vi "pid-tuning-v2.vi"() -> ()   [LabVIEW 2019]
uses:
  <vilib>/DAQmx/read.llb/DAQmx Read (Analog 1D DBL 1Chan NSamp).vi
  <vilib>/Analysis/baseanly.llb/Mean (DBL).vi
  <vilib>/DAQmx/write.llb/DAQmx Write (Analog DBL 1Chan 1Samp).vi
  <vilib>/DAQmx/create/channels.llb/DAQmx Create Channel (AO-Current-Basic).vi
  <vilib>/DAQmx/create/channels.llb/DAQmx Create Channel (AI-Current-Basic).vi
  <vilib>/DAQmx/miscellaneous.llb/DAQmx Fill In Error Info.vi
  <vilib>/Analysis/NI_AALBase.lvlib
  <vilib>/addons/control/pid/NI_PID_autopid.lvlib
panel:
  out "PID FINAL POWER":dbl
  in  "stop":bool
  out "PID START TIME":dbl
  in  "Tabs":T1(tab)
  in  "POWER CONTROL":dbl format="%#_13g"
  in  "ENABLE FURNACE TEST":bool[](array[boolean])=[FALSE]
  in  "STOP FURNACE TEST":bool[](array[boolean])=[FALSE]
  in  "Close Valve":bool[](array[boolean])=[TRUE]
  in  "Purge Flow":bool[](array[boolean])=[FALSE]
  in  "ARGON OUT 0-.02":dbl format="%#_13g"
  out "VALVE OUTPUT":dbl
  out "PYROMETER TEMP":dbl
  out "PYROMETER READING":dbl
  in  "RAMP UP POWER":dbl format="%#_13g"
  out "TEMPERATURE OVER TIME":cluster{dbl[], dbl[]}[](graph)
  out "CURRENT TEMPERATURE (C)":dbl
  in  "PID SETPOINT":dbl=820.0
  in  "Clear Data":bool
  in  "Restart PID":bool
  in  "PID gains":T2={"proportional gain (Kc)"=5e-05, "integral time (Ti, min)"=1.5, "derivative time (Td, min)"=0.0} {"derivative time (Td, min)" format="%.8f"; "integral time (Ti, min)" format="%.24f"; "proportional gain (Kc)" format="%.8f"}
  out "POWER LEVEL OUTPUT (%)":dbl
  out "tuning completed?":bool
  in  "autotune? (F)":bool
  out "PID gains out":T2={"proportional gain (Kc)"=1.0, "integral time (Ti, min)"=0.01, "derivative time (Td, min)"=0.0} {"derivative time (Td, min)" format="%.3f"; "integral time (Ti, min)" format="%.3f"; "proportional gain (Kc)" format="%.3f"}
  out "Time has Elapsed 2":bool caption="Time has Elapsed"
  out "CURRENT RAMP DOWN POWER LEVEL":string
  out "PYROMETER READING 2":dbl
  in  "RAMP DOWN TIME (min)":dbl=10.0
  in  "Mode":T3(ring)
  in  "POWER OUT":dbl format="%#_13g"
  in  "STOP FURNACE":bool[](array[boolean])
  in  "ENABLE FURNACE":bool[](array[boolean])
  out "DONE":bool
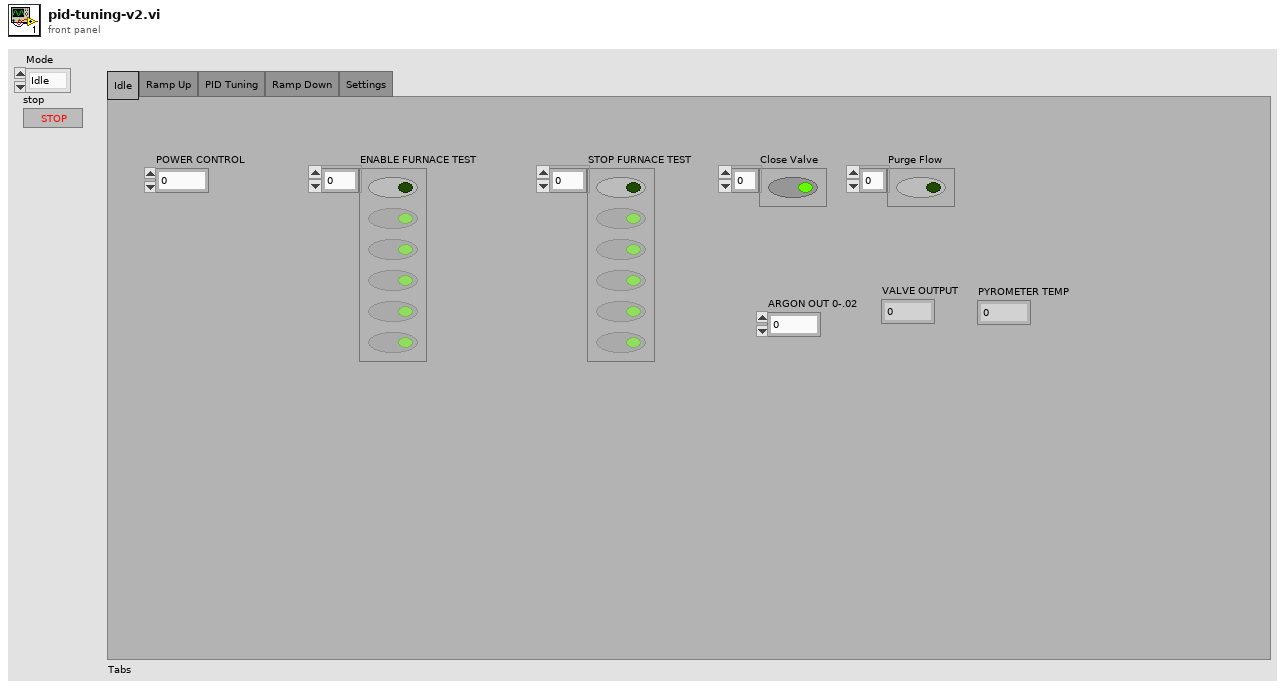
[diagram p1: front panel]
types:
  T1 = enum32{"Idle", "Ramp Up", "PID Tuning", "Ramp Down", "Settings"}
  T2 = cluster{"proportional gain (Kc)":dbl, "integral time (Ti, min)":dbl, "derivative time (Td, min)":dbl}
  T3 = enum16{"Idle", "Ramp Up", "PID Tune", "Ramp Down"}
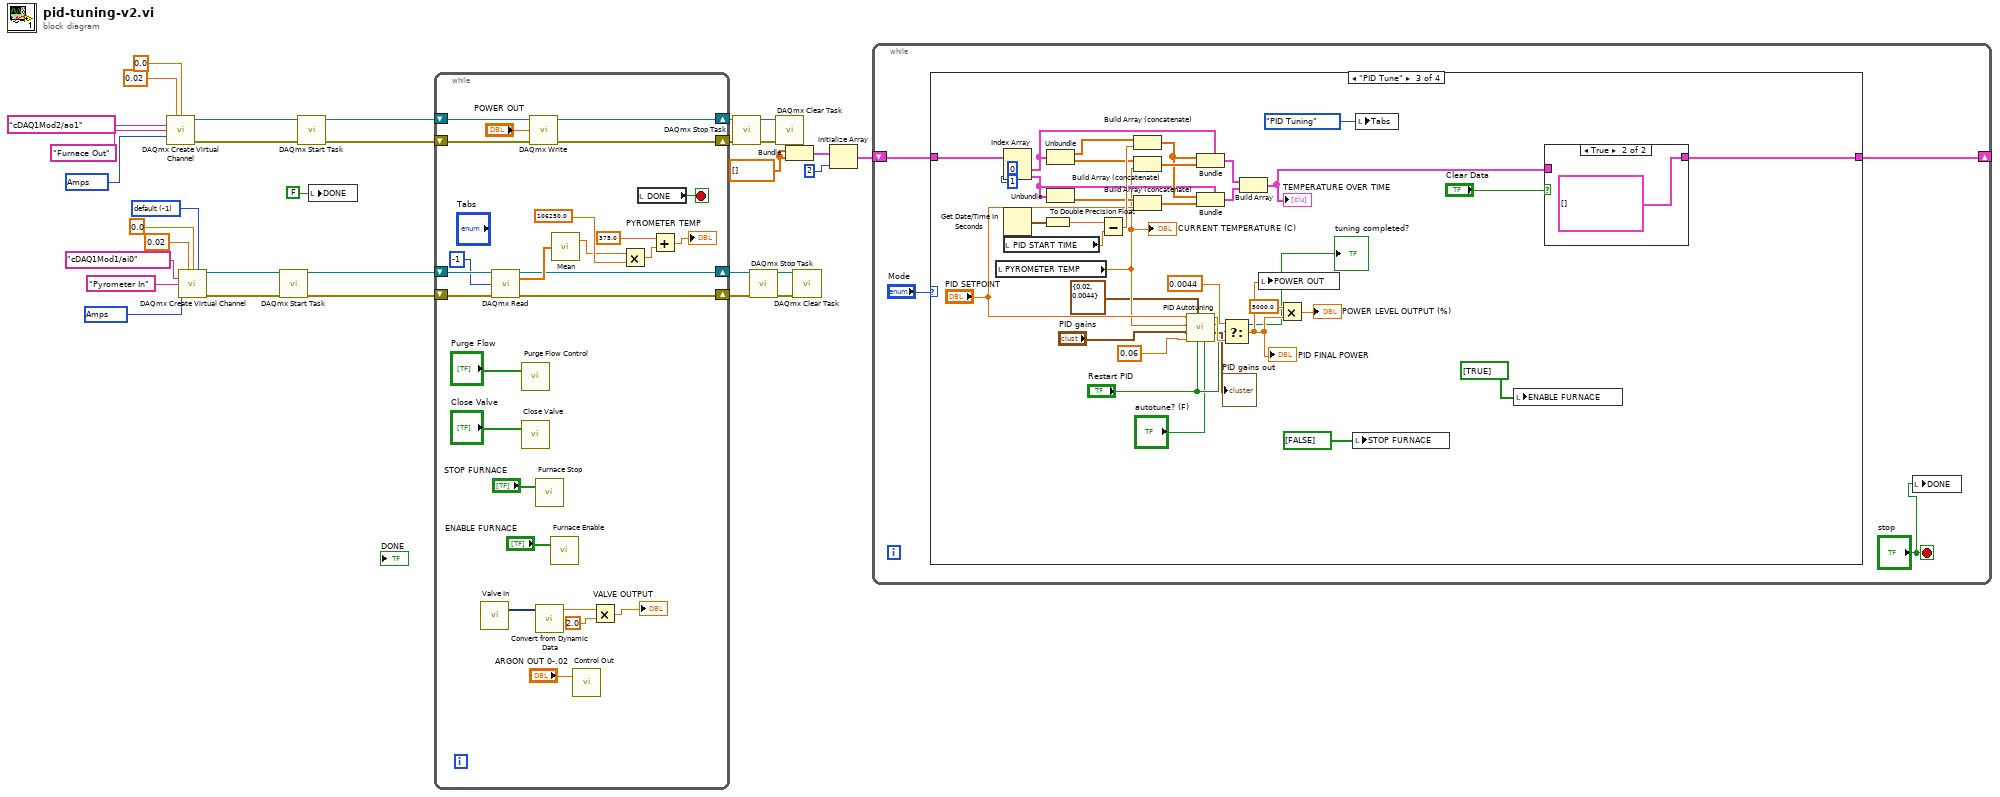
[diagram p0: block diagram]
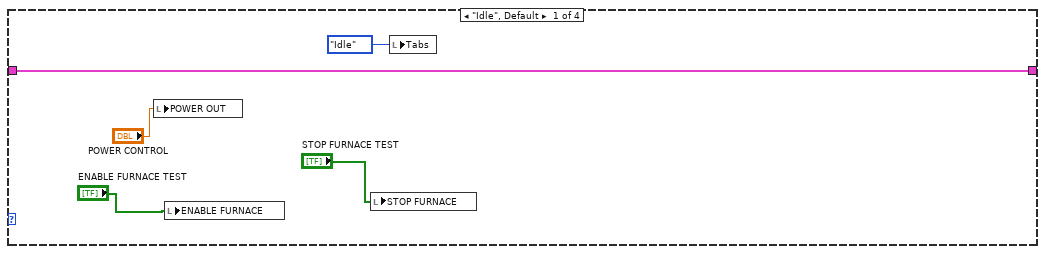
[diagram p2: hidden frame]
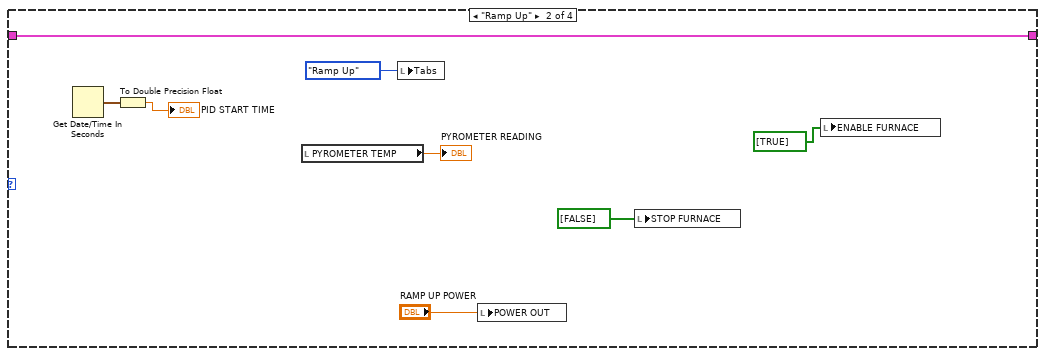
[diagram p3: hidden frame]
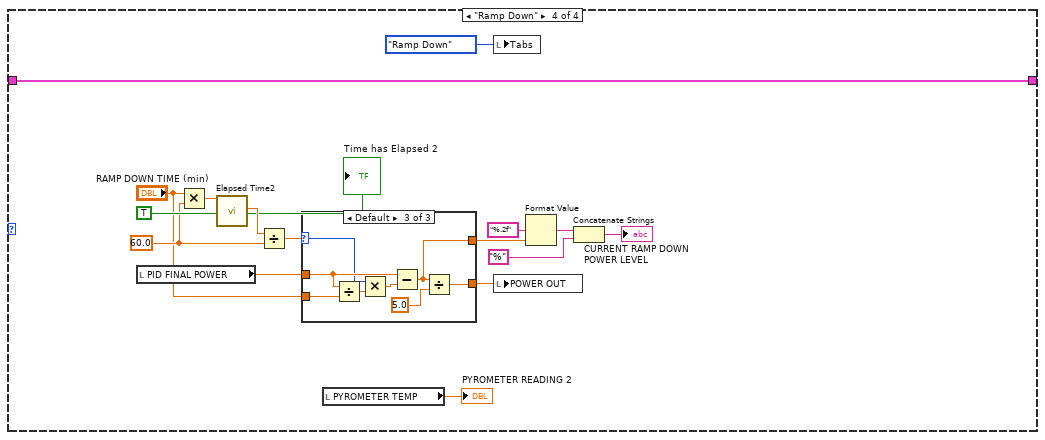
[diagram p5: hidden frame]
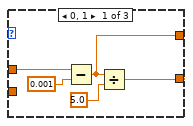
[diagram p6: hidden frame]
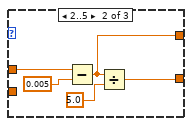
[diagram p7: hidden frame]
diagram:
  w9 = -1 items=["default"=-1, "RSE"=10083, "NRSE"=10078, "Differential"=10106, "Pseudodifferential"=12529] ("input terminal configuration")
  w10 = 10342 items=["Amps"=10342, "From Custom Scale"=10065] ("units")
  w26 = 10342 items=["Amps"=10342, "From Custom Scale"=10065] ("units")
  w31 = dbl[] []
  n1 = call-poly <vilib>:"DAQmx Create Virtual Channel.vi"("maximum value"=0.02, "minimum value"=0.0, "physical channels"=tag "cDAQ1Mod2/ao1", "name to assign"="Furnace Out", "units"=w26) -> ("task out"=w17:refnum<k21>, "error out"=w16:errorcluster)  [unwired: 9 in]
  n2 = call-poly <vilib>:"DAQmx Create Virtual Channel.vi"("maximum value"=0.02, "minimum value"=0.0, "input terminal configuration"=w9, "physical channels"=tag "cDAQ1Mod1/ai0", "name to assign"="Pyrometer In", "units"=w10) -> ("task out"=w8:refnum<k21>, "error out"=w7:errorcluster)  [unwired: 8 in]
  n3 = call <vilib>:"DAQmx Start Task.vi"("task/channels in"=w8, "error in"=w7) -> ("task out"=w6:refnum<k21>, "error out"=w5:errorcluster)  [unwired: 12 in]
  n4 = call <vilib>:"DAQmx Start Task.vi"("task/channels in"=w17, "error in"=w16) -> ("task out"=w19:refnum<k21>, "error out"=w18:errorcluster)  [unwired: 12 in]
  n5 = local write "DONE"(FALSE ("DONE")) -> ()
  n6 = while {
    shift-right: [w48] -> w23
    shift-left: w19 -> [w51]
    shift-right: [w47] -> w22
    shift-left: w18 -> [w50]
    shift-right: [w40] -> w3
    shift-left: w6 -> [w44]
    shift-right: [w39] -> w2
    shift-left: w5 -> [w42]
    stop <- w58 stop-if-true
    n7 = call "Valve In"() -> ("data"=w37:dynamicdata)  [unwired: 16 in, 3 out]
    n8 = call-poly <vilib>:"DAQmx Read.vi"("task/channels in"=w44, "number of samples per channel"=-1, "error in"=w42) -> ("task out"=w40:refnum<k21>, "data"=w41:dbl[], "error out"=w39:errorcluster)  [unwired: 10 in]
    n9 = call "Purge Flow Control"("data"="Purge Flow") -> ()  [unwired: 17 in, 2 out]
    n10 = call "Close Valve"("data"="Close Valve") -> ()  [unwired: 17 in, 2 out]
    n11 = call-poly <vilib>:"DAQmx Write.vi"("task/channels in"=w51, "data"="POWER OUT", "error in"=w50) -> ("task out"=w48:refnum<k21>, "error out"=w47:errorcluster)  [unwired: 10 in, 1 out]
    n12 = call "Furnace Stop"("data"="STOP FURNACE") -> ()  [unwired: 17 in, 2 out]
    n13 = call "Convert from Dynamic Data"("Dynamic Data Type"=w37) -> ("Scalar"=w36:dbl)  [unwired: 3 in]
    n14 = call "Furnace Enable"("data"="ENABLE FURNACE") -> ()  [unwired: 17 in, 2 out]
    n15 = call-poly <vilib>:"Mean.vi"("X"=w41) -> ("mean"=w45:dbl)  [unwired: 1 out]
    n16 = call "Control Out"("data"="ARGON OUT 0-.02") -> ()  [unwired: 17 in, 2 out]
    n17 = Multiply(x=w36, y=2.0) -> (x*y=→"VALVE OUTPUT":dbl)
    n18 = Multiply(x=w45, y=106250.0) -> (x*y=w54:dbl)
    n19 = local read "DONE"() -> (w58:bool)
    n20 = Add(x=375.0, y=w54) -> (x+y=→"PYROMETER TEMP":dbl)
  }
  n21 = call <vilib>:"DAQmx Stop Task.vi"("task/channels in"=w23, "error in"=w22) -> ("task out"=w21:refnum<k21>, "error out"=w20:errorcluster)  [unwired: 12 in]
  n22 = call <vilib>:"DAQmx Stop Task.vi"("task/channels in"=w3, "error in"=w2) -> ("task out"=w4:refnum<k21>, "error out"=w1:errorcluster)  [unwired: 12 in]
  n23 = call <vilib>:"DAQmx Clear Task.vi"("task in"=w21, "error in"=w20) -> ()  [unwired: 13 in, 1 out]
  n24 = Bundle(w31, w31) -> (w32:cluster{dbl[], dbl[]})  [unwired: 1 in]
  n25 = call <vilib>:"DAQmx Clear Task.vi"("task in"=w4, "error in"=w1) -> ()  [unwired: 13 in, 1 out]
  n26 = Initialize Array(w32, 2 ("dimension size")) -> (w29:cluster{dbl[], dbl[]}[])
  n27 = while {
    shift-right: [w60] -> _
    shift-left: w29 -> [w61]
    stop <- "stop" stop-if-true
    n28 = case shown="\"PID Tune\"" "Mode" {
      tunnel: w61 -> [w66 w71 w96 w118]
      tunnel: [w66 w71 w93 w118] -> w60
      frame "Idle", Default {
        n29 = local write "POWER OUT"("POWER CONTROL") -> ()
        n30 = local write "ENABLE FURNACE"("ENABLE FURNACE TEST") -> ()
        n31 = local write "STOP FURNACE"("STOP FURNACE TEST") -> ()
        n32 = local write "Tabs"(T1."Idle" ("Tabs")) -> ()
      }
      frame "Ramp Up" {
        n33 = Get Date/Time In Seconds() -> (seconds since 1Jan1904=w70:timestamp)
        n34 = To Double Precision Float(number=w70) -> (double precision float=→"PID START TIME":dbl)
        n35 = local read "PYROMETER TEMP"() -> (→"PYROMETER READING":dbl)
        n36 = local write "Tabs"(T1."Ramp Up" ("Tabs")) -> ()
        n37 = local write "POWER OUT"("RAMP UP POWER") -> ()
        n38 = local write "STOP FURNACE"(bool[] [FALSE] ("ENABLE FURNACE")) -> ()
        n39 = local write "ENABLE FURNACE"(bool[] [TRUE] ("Boolean")) -> ()
      }
      frame "PID Tune" {
        n40 = local read "PYROMETER TEMP"() -> (w84:dbl)
        "CURRENT TEMPERATURE (C)" <- w84
        n41 = Index Array(array=w96, index #1=0 ("index"), index #2=1 ("index")) -> (element #1=w107:cluster{dbl[], dbl[]}, element #2=w99:cluster{dbl[], dbl[]})
        n42 = Get Date/Time In Seconds() -> (seconds since 1Jan1904=w112:timestamp)
        n43 = local read "PID START TIME"() -> (w110:dbl)
        n44 = To Double Precision Float(number=w112) -> (double precision float=w111:dbl)
        n45 = Unbundle(w107) -> (w106:dbl[], w104:dbl[])
        n46 = Unbundle(w99) -> (w103:dbl[])  [unwired: 1 out]
        n47 = Subtract(x=w111, y=w110) -> (x-y=w105:dbl)
        n48 = Build Array (concatenate)(w106, w105) -> (w101:dbl[])
        n49 = Build Array (concatenate)(w104, w84) -> (w102:dbl[])
        n50 = Build Array (concatenate)(w103, "PID SETPOINT") -> (w100:dbl[])
        n51 = call <vilib>:"PID Autotuning.vi"("autotune? (F)"="autotune? (F)", "reinitialize? (F)"="Restart PID", "output range"=cluster{"output high":dbl, "output low":dbl} {"output high"=0.02, "output low"=0.0044}, "dt (s)"=0.06, "PID gains"="PID gains", "process variable"=w84, "setpoint"="PID SETPOINT") -> ("PID gains out"=→"PID gains out":T2, "tuning completed?"=→"tuning completed?":bool, "output"=w81:dbl)  [unwired: 1 in, 1 out]
        n52 = Bundle(cluster=w107, w101, w102) -> (w97:cluster{dbl[], dbl[]})
        n53 = Bundle(cluster=w99, w101, w100) -> (w98:cluster{dbl[], dbl[]})
        n54 = Select(t=0.0044, s="Restart PID", f=w81) -> (s? t:f=w86:dbl)
        "PID FINAL POWER" <- w86
        n55 = Build Array(w97, w98) -> (w94:cluster{dbl[], dbl[]}[])
        "TEMPERATURE OVER TIME" <- w94
        n56 = local write "POWER OUT"(w86) -> ()
        n57 = Multiply(x=5000.0 ("y"), y=w86) -> (x*y=→"POWER LEVEL OUTPUT (%)":dbl)
        n58 = local write "STOP FURNACE"(bool[] [FALSE] ("ENABLE FURNACE")) -> ()
        n59 = local write "Tabs"(T1."PID Tuning" ("Tabs")) -> ()
        n60 = local write "ENABLE FURNACE"(bool[] [TRUE] ("Boolean")) -> ()
        n61 = case shown="True" "Clear Data" {
          tunnel: w94 -> [w113 _]
          tunnel: [w113 cluster{dbl[], dbl[]}[] []] -> w93
          frame False {
          }
          frame True {
          }
        }
      }
      frame "Ramp Down" {
        w128 = 60.0 ("y")
        n62 = local read "PID FINAL POWER"() -> (w126:dbl)
        n63 = Multiply(x="RAMP DOWN TIME (min)", y=w128) -> (x*y=w130:dbl)
        n64 = call "Elapsed Time2"("Time Target (s)"=w130, "Auto Reset"=TRUE) -> ("Elapsed Time (s)"=w129:dbl, "Time has Elapsed"=→"Time has Elapsed 2":bool)  [unwired: 10 in, 6 out]
        n65 = Divide(x=w129, y=w128) -> (x/y=w127:dbl)
        n66 = case shown="Default" w127 {
          selector: w127 -> [_ _ w146]
          tunnel: w126 -> [w136 w139 w149]
          tunnel: [w133 w138 w143] -> w125
          tunnel: "RAMP DOWN TIME (min)" -> [_ _ w148]
          tunnel: [w132 w137 w142] -> w120
          frame 0, 1 {
            n67 = Subtract(x=w136, y=0.001) -> (x-y=w132:dbl)
            n68 = Divide(x=w132, y=5.0) -> (x/y=w133:dbl)
          }
          frame 2..5 {
            n69 = Subtract(x=w139, y=0.005) -> (x-y=w137:dbl)
            n70 = Divide(x=w137, y=5.0) -> (x/y=w138:dbl)
          }
          frame Default {
            n71 = Divide(x=w149, y=w148) -> (x/y=w147:dbl)
            n72 = Multiply(x=w146, y=w147) -> (x*y=w145:dbl)
            n73 = Subtract(x=w149, y=w145) -> (x-y=w142:dbl)
            n74 = Divide(x=w142, y=5.0) -> (x/y=w143:dbl)
          }
        }
        n75 = local read "PYROMETER TEMP"() -> (→"PYROMETER READING 2":dbl)
        n76 = local write "Tabs"(T1."Ramp Down" ("Tabs")) -> ()
        n77 = local write "POWER OUT"(w125) -> ()
        n78 = Format Value(format string="%.2f", value (0)=w120) -> (output string=w123:string)  [unwired: 1 in]
        n79 = Concatenate Strings(w123, "%" ("format string")) -> (→"CURRENT RAMP DOWN POWER LEVEL":string)
      }
    }
    n80 = local write "DONE"("stop") -> ()
  }
